vi "import matrix.vi"() -> (3 "String Array From File":string[][](array[string]))   [LabVIEW 2017]
uses:
  <vilib>/Utility/file.llb/Read Delimited Spreadsheet (string).vi
panel:
  in  "Search String":string
  out "Check Array":dbl[](array[numeric])
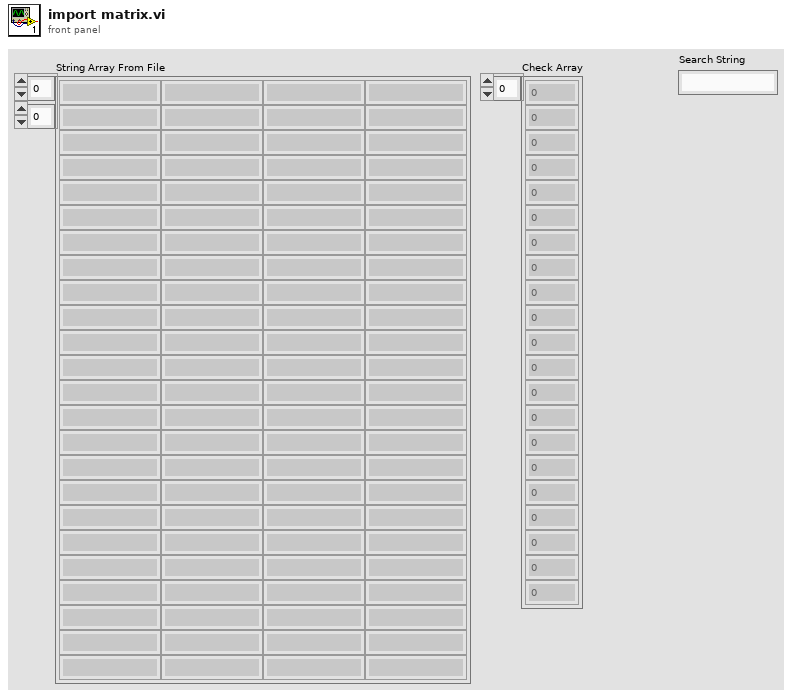
[diagram p1: front panel]
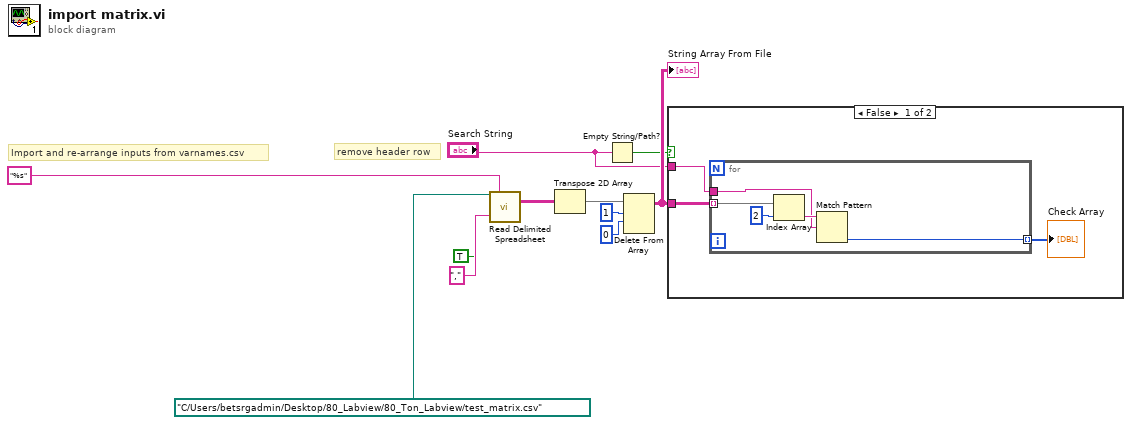
[diagram p0: block diagram]
diagram:
  # "remove header row"
  # "Import and re-arrange inputs from varnames.csv"
  n1 = call-poly <vilib>:"Read Delimited Spreadsheet.vi"("file path (dialog if empty)"=path "C:/Users/betsrgadmin/Desktop/80_Labview/80_Ton_Labview/test_matrix.csv", "format (%s)"="%s", "transpose? (F)"=TRUE, "delimiter (\\t)"=",") -> ("all rows"=w8:string[][])  [unwired: 6 in, 5 out]
  n2 = Transpose 2D Array(2D array=w8) -> (transposed array=w7:string[][])
  n3 = Empty String/Path?(string/path="Search String") -> (empty?=w3:bool)
  n4 = Delete From Array(array=w7, length=1, index (row)=0) -> (array with subset deleted=w4:string[][])  [unwired: 1 in, 1 out]
  "String Array From File" <- w4
  n5 = case shown="False" w3 {
    tunnel: w4 -> [w13 _]
    tunnel: "Search String" -> [w12 _]
    frame False {
      n6 = for {
        tunnel: w13 -> [w19] mode=indexing
        tunnel: [w17] -> w14 mode=indexing
        tunnel: w12 -> [w15]
        n7 = Index Array(array=w19, index=2) -> (element=w18:string)
        n8 = Match Pattern(string=w18, regular expression=w15) -> (offset past match=w17:i32)  [unwired: 1 in, 3 out]
      }
      "Check Array" <- w14
    }
    frame True {
    }
  }
